vi "Homework_Files.vi"() -> ()   [LabVIEW 2021]
uses:
  <vilib>/numeric/Random Number (Range) DBL.vi
panel:
  in  "stop":bool
  out "XY Graph":cluster{i32[], dbl[]}[](graph)
  out "text":string
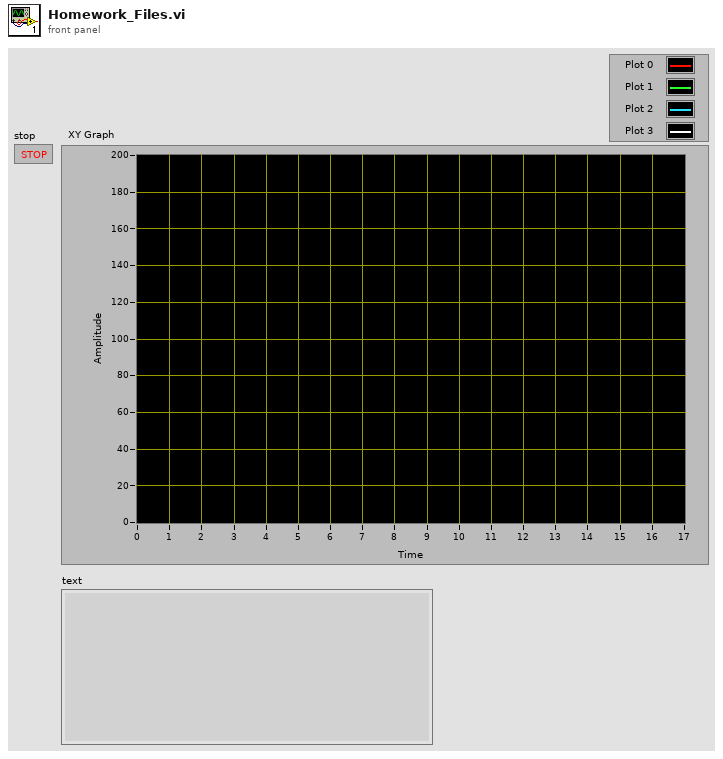
[diagram p1: front panel]
types:
  T1 = enum16{"open", "replace", "create", "open or create", "replace or create", "replace or create with confirmation"}
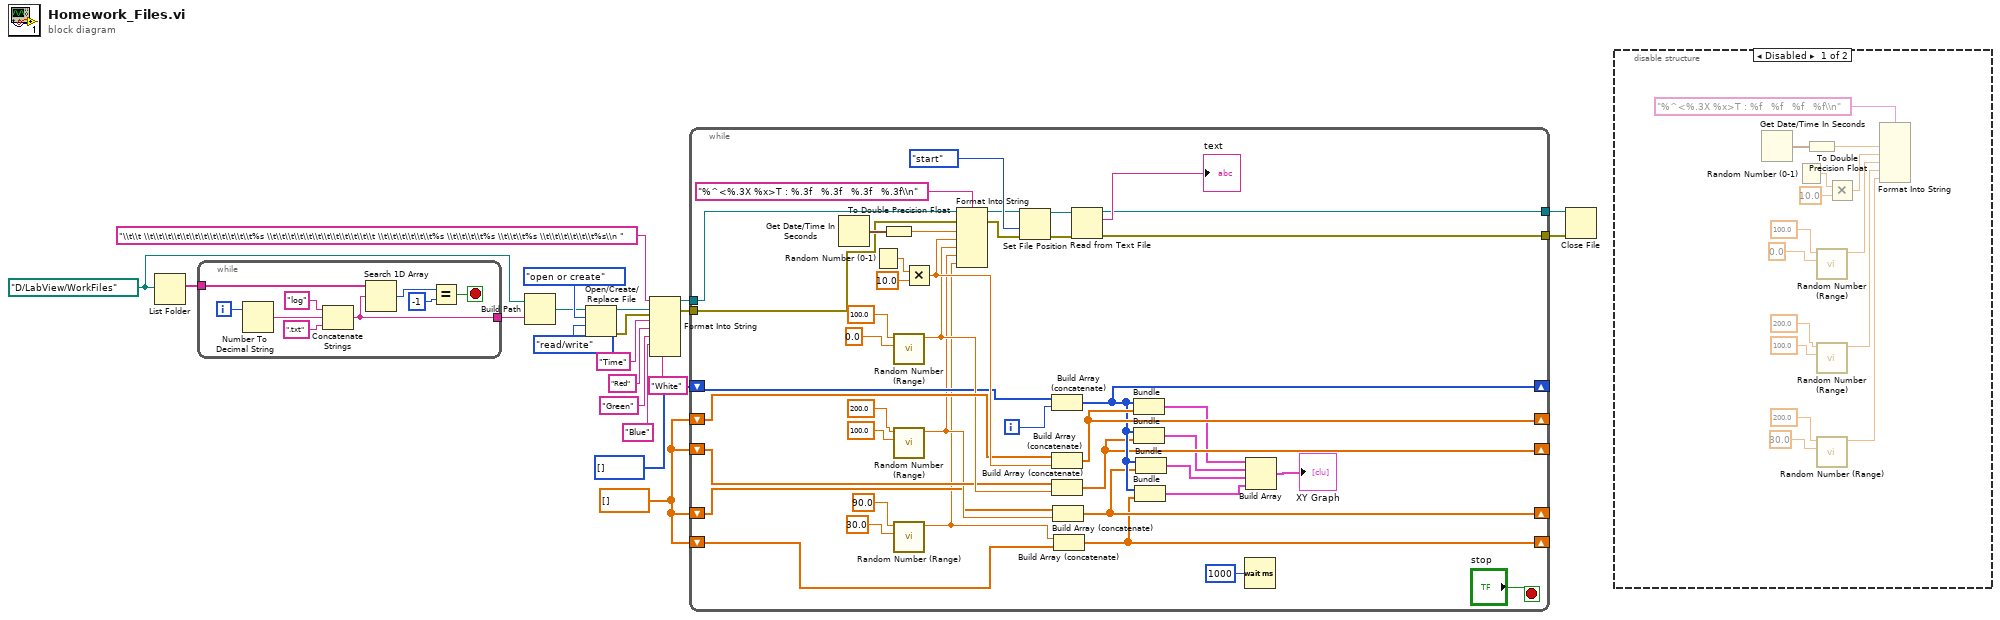
[diagram p0: block diagram]
diagram:
  w1 = dbl[] []
  w18 = path "D:/LabView/WorkFiles" ("file path (use dialog)")
  n1 = List Folder(path=w18) -> (filenames=w20:string[])  [unwired: 3 in, 3 out]
  n2 = while {
    tunnel: w20 -> [w29]
    tunnel: [w22] -> w19
    i -> [w21]
    stop <- w26 stop-if-true
    n3 = Number To Decimal String(number=w21) -> (decimal integer string=w24:string)  [unwired: 1 in]
    n4 = Concatenate Strings("log", w24, ".txt") -> (w22:string)
    n5 = Search 1D Array(1D array=w29, element=w22) -> (index of element=w28:i32)  [unwired: 1 in]
    n6 = Equal?(x=w28, y=-1) -> (x = y?=w26:bool)
  }
  n7 = Build Path(base path=w18, name or relative path=w19) -> (appended path=w15:path)
  n8 = Open/Create/Replace File(file path (use dialog)=w15, operation (0:open)=T1."open or create", access (0:read/write)=enum16{"read/write", "read-only", "write-only"}."read/write") -> (refnum out=w14:refnum<file>, error out=w7:errorcluster)  [unwired: 3 in, 1 out]
  n9 = Format Into String(format string="\\t\\t \\t\\t\\t\\t\\t\\t\\t\\t\\t\\t\\t\\t%s \\t\\t\\t\\t\\t\\t\\t\\t\\t\\t\\t\\t \\t\\t\\t\\t\\t\\t%s \\t\\t\\t\\t%s \\t\\t\\t%s \\t\\t\\t\\t\\t\\t%s\\n ", initial string=w14, error in=w7, "Time" ("input 1"), "Red" ("input 2"), "Green" ("input 3"), "Blue" ("input 4"), "White" ("input 5")) -> (resulting string=w6:refnum<file>, error out=w5:errorcluster)
  n10 = while {
    tunnel: w6 -> [w61]
    tunnel: w5 -> [w60]
    shift-right: [w50] -> _
    shift-left: w1 -> [w51]
    tunnel: [w48] -> w4
    tunnel: [w47] -> w3
    shift-right: [w44] -> _
    shift-left: w1 -> [w46]
    shift-right: [w45] -> _
    shift-left: i32[] [] -> [w43]
    shift-right: [w39] -> _
    shift-left: w1 -> [w40]
    shift-right: [w36] -> _
    shift-left: w1 -> [w38]
    i -> [w53]
    stop <- "stop" stop-if-true
    n11 = Get Date/Time In Seconds() -> (seconds since 1Jan1904=w71:timestamp)
    n12 = Random Number (0-1)() -> (number: 0 to 1=w70:dbl)
    n13 = To Double Precision Float(number=w71) -> (double precision float=w72:dbl)
    n14 = call-poly <vilib>:"Random Number (Range).vi"("lower bound (0)"=0.0, "upper bound (100)"=100.0) -> ("number"=w49:dbl)  [unwired: 9 in]
    n15 = call-poly <vilib>:"Random Number (Range).vi"("lower bound (0)"=100.0, "upper bound (100)"=200.0) -> ("number"=w41:dbl)  [unwired: 9 in]
    n16 = call-poly <vilib>:"Random Number (Range).vi"("lower bound (0)"=30.0, "upper bound (100)"=90.0) -> ("number"=w37:dbl)  [unwired: 9 in]
    n17 = Multiply(x=w70, y=10.0) -> (x*y=w52:dbl)
    n18 = Format Into String(format string="%^<%.3X %x>T : %.3f   %.3f   %.3f   %.3f\\n", initial string=w61, error in=w60, w72, w52, w49, w41, w37) -> (resulting string=w54:refnum<file>, error out=w59:errorcluster)
    n19 = Set File Position(refnum=w54, from (0:start)=enum16{"start", "end", "current"}."start", error in=w59) -> (refnum out=w56:refnum<file>, error out=w55:errorcluster)  [unwired: 1 in]
    n20 = Build Array (concatenate)(w43, w53) -> (w45:i32[])
    n21 = Build Array (concatenate)(w51, w52) -> (w50:dbl[])
    n22 = Build Array (concatenate)(w46, w49) -> (w44:dbl[])
    n23 = Build Array (concatenate)(w40, w41) -> (w39:dbl[])
    n24 = Build Array (concatenate)(w37, w38) -> (w36:dbl[])
    n25 = Read from Text File(file (use dialog)=w56, error in=w55) -> (refnum out=w47:refnum<file>, text=→"text":string, error out=w48:errorcluster)  [unwired: 2 in, 1 out]
    n26 = Bundle(w45, w50) -> (w35:cluster{i32[], dbl[]})  [unwired: 1 in]
    n27 = Bundle(w45, w44) -> (w34:cluster{i32[], dbl[]})  [unwired: 1 in]
    n28 = Bundle(w45, w36) -> (w32:cluster{i32[], dbl[]})  [unwired: 1 in]
    n29 = Bundle(w45, w39) -> (w33:cluster{i32[], dbl[]})  [unwired: 1 in]
    n30 = Wait (ms)(milliseconds to wait=u32 1000) -> ()  [unwired: 1 out]
    n31 = Build Array(w35, w34, w33, w32) -> (→"XY Graph":cluster{i32[], dbl[]}[])
  }
  n32 = Close File(refnum=w3, error in=w4) -> ()  [unwired: 2 out]
  n33 = disable-structure shown="Disabled" {
    frame Disabled {
      n34 = Get Date/Time In Seconds() -> (seconds since 1Jan1904=w85:timestamp)
      n35 = Random Number (0-1)() -> (number: 0 to 1=w84:dbl)
      n36 = To Double Precision Float(number=w85) -> (double precision float=w86:dbl)
      n37 = call-poly <vilib>:"Random Number (Range).vi"("lower bound (0)"=0.0, "upper bound (100)"=100.0) -> ("number"=w83:dbl)  [unwired: 9 in]
      n38 = call-poly <vilib>:"Random Number (Range).vi"("lower bound (0)"=100.0, "upper bound (100)"=200.0) -> ("number"=w82:dbl)  [unwired: 9 in]
      n39 = call-poly <vilib>:"Random Number (Range).vi"("lower bound (0)"=30.0, "upper bound (100)"=200.0) -> ("number"=w81:dbl)  [unwired: 9 in]
      n40 = Multiply(x=w84, y=10.0) -> (x*y=w87:dbl)
      n41 = Format Into String(format string="%^<%.3X %x>T : %f   %f   %f   %f\\n", w86, w87, w83, w82, w81) -> ()  [unwired: 2 in, 2 out]
    }
    frame Enabled {
    }
  }
